vi "报文解析.vi"(9 "长度":i32, 10 "起始位":i32, 11 "MessageBuffer in":T1 {"DATA"."[0]" format="%x"; "DATA"."[1]" format="%x"; "DATA"."[2]" format="%x"; "DATA"."[3]" format="%x"; "DATA"."[4]" format="%x"; "DATA"."[5]" format="%x"; "DATA"."[6]" format="%x"; "DATA"."[7]" format="%x"; "DATA"."[8]" format="%x"; "DATA"."[9]" format="%x"; "DATA"."[10]" format="%x"; "DATA"."[11]" format="%x"; "DATA"."[12]" format="%x"; "DATA"."[13]" format="%x"; "DATA"."[14]" format="%x"; "DATA"."[15]" format="%x"; "DATA"."[16]" format="%x"; "DATA"."[17]" format="%x"; "DATA"."[18]" format="%x"; "DATA"."[19]" format="%x"; "DATA"."[20]" format="%x"; "DATA"."[21]" format="%x"; "DATA"."[22]" format="%x"; "DATA"."[23]" format="%x"; "DATA"."[24]" format="%x"; "DATA"."[25]" format="%x"; "DATA"."[26]" format="%x"; "DATA"."[27]" format="%x"; "DATA"."[28]" format="%x"; "DATA"."[29]" format="%x"; "DATA"."[30]" format="%x"; "DATA"."[31]" format="%x"; "DATA"."[32]" format="%x"; "DATA"."[33]" format="%x"; "DATA"."[34]" format="%x"; "DATA"."[35]" format="%x"; "DATA"."[36]" format="%x"; "DATA"."[37]" format="%x"; "DATA"."[38]" format="%x"; "DATA"."[39]" format="%x"; "DATA"."[40]" format="%x"; "DATA"."[41]" format="%x"; "DATA"."[42]" format="%x"; "DATA"."[43]" format="%x"; "DATA"."[44]" format="%x"; "DATA"."[45]" format="%x"; "DATA"."[46]" format="%x"; "DATA"."[47]" format="%x"; "DATA"."[48]" format="%x"; "DATA"."[49]" format="%x"; "DATA"."[50]" format="%x"; "DATA"."[51]" format="%x"; "DATA"."[52]" format="%x"; "DATA"."[53]" format="%x"; "DATA"."[54]" format="%x"; "DATA"."[55]" format="%x"; "DATA"."[56]" format="%x"; "DATA"."[57]" format="%x"; "DATA"."[58]" format="%x"; "DATA"."[59]" format="%x"; "DATA"."[60]" format="%x"; "DATA"."[61]" format="%x"; "DATA"."[62]" format="%x"; "DATA"."[63]" format="%x"; "ID" format="%.0x"; "MSGTYPE" format="%.0x"; "DLC" format="%.0x"}) -> (3 "数字":u32)   [LabVIEW 2020]
uses:
  <userlib>/PCANBasic/ctl/TPCANMsgFD.ctl
  <userlib>/PCANBasic/PCANBasic.lvlib
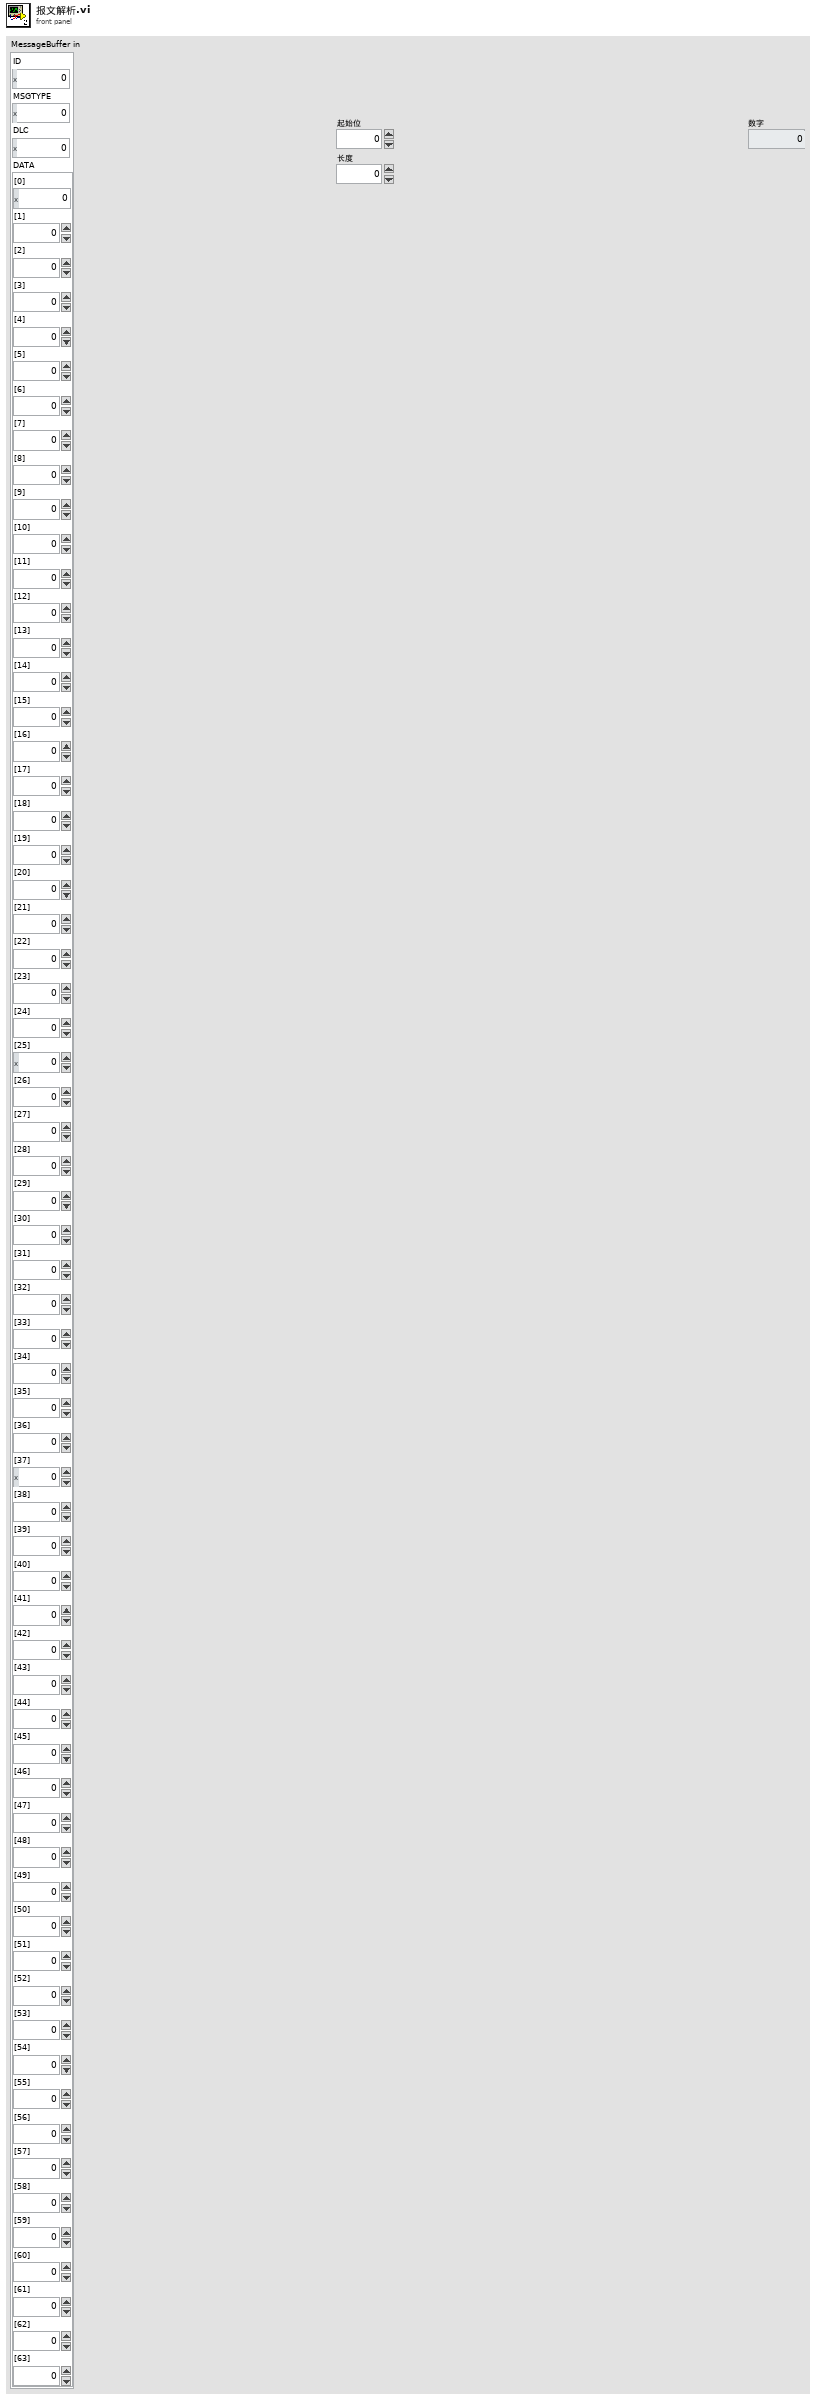
[diagram p1: front panel]
types:
  T1 = typedef "PCANBasic.lvlib/TPCANMsgFD.ctl" = cluster{"ID":u32, "MSGTYPE":u8, "DLC":u8, "DATA":cluster{"[0]":u8, "[1]":u8, "[2]":u8, "[3]":u8, "[4]":u8, "[5]":u8, "[6]":u8, "[7]":u8, "[8]":u8, "[9]":u8, "[10]":u8, "[11]":u8, "[12]":u8, "[13]":u8, "[14]":u8, "[15]":u8, "[16]":u8, "[17]":u8, "[18]":u8, "[19]":u8, "[20]":u8, "[21]":u8, "[22]":u8, "[23]":u8, "[24]":u8, "[25]":u8, "[26]":u8, "[27]":u8, "[28]":u8, "[29]":u8, "[30]":u8, "[31]":u8, "[32]":u8, "[33]":u8, "[34]":u8, "[35]":u8, "[36]":u8, "[37]":u8, "[38]":u8, "[39]":u8, "[40]":u8, "[41]":u8, "[42]":u8, "[43]":u8, "[44]":u8, "[45]":u8, "[46]":u8, "[47]":u8, "[48]":u8, "[49]":u8, "[50]":u8, "[51]":u8, "[52]":u8, "[53]":u8, "[54]":u8, "[55]":u8, "[56]":u8, "[57]":u8, "[58]":u8, "[59]":u8, "[60]":u8, "[61]":u8, "[62]":u8, "[63]":u8}}
  T2 = cluster{"[0]":u8, "[1]":u8, "[2]":u8, "[3]":u8, "[4]":u8, "[5]":u8, "[6]":u8, "[7]":u8, "[8]":u8, "[9]":u8, "[10]":u8, "[11]":u8, "[12]":u8, "[13]":u8, "[14]":u8, "[15]":u8, "[16]":u8, "[17]":u8, "[18]":u8, "[19]":u8, "[20]":u8, "[21]":u8, "[22]":u8, "[23]":u8, "[24]":u8, "[25]":u8, "[26]":u8, "[27]":u8, "[28]":u8, "[29]":u8, "[30]":u8, "[31]":u8, "[32]":u8, "[33]":u8, "[34]":u8, "[35]":u8, "[36]":u8, "[37]":u8, "[38]":u8, "[39]":u8, "[40]":u8, "[41]":u8, "[42]":u8, "[43]":u8, "[44]":u8, "[45]":u8, "[46]":u8, "[47]":u8, "[48]":u8, "[49]":u8, "[50]":u8, "[51]":u8, "[52]":u8, "[53]":u8, "[54]":u8, "[55]":u8, "[56]":u8, "[57]":u8, "[58]":u8, "[59]":u8, "[60]":u8, "[61]":u8, "[62]":u8, "[63]":u8}
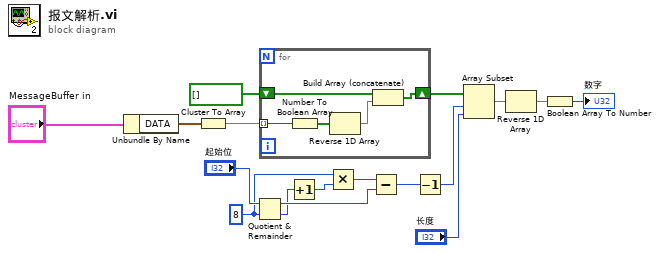
[diagram p0: block diagram]
diagram:
  w6 = 8 ("y")
  n1 = Unbundle By Name("MessageBuffer in") -> ("DATA"=w2:T2)
  n2 = Cluster To Array(cluster=w2) -> (array=w1:u8[])
  n3 = Quotient & Remainder(x="起始位", y=w6) -> (x-y*floor(x/y)=w9:i32, floor(x/y)=w7:i32)
  n4 = for {
    shift-right: [w22] -> w16
    shift-left: bool[] [] -> [w21]
    tunnel: w1 -> [w18] mode=indexing
    n5 = Number To Boolean Array(number=w18) -> (Boolean array=w20:bool[])
    n6 = Reverse 1D Array(array=w20) -> (reversed array=w19:bool[])
    n7 = Build Array (concatenate)(w21, w19) -> (w22:bool[])
  }
  n8 = Increment(x=w7) -> (x+1=w8:i32)
  n9 = Multiply(x=w6, y=w8) -> (x*y=w10:i32)
  n10 = Subtract(x=w10, y=w9) -> (x-y=w5:i32)
  n11 = Decrement(x=w5) -> (x-1=w4:i32)
  n12 = Array Subset(array=w16, index=w4, length="长度") -> (w13:bool[])
  n13 = Reverse 1D Array(array=w13) -> (reversed array=w12:bool[])
  n14 = Boolean Array To Number(Boolean array=w12) -> (number=→"数字":u32)
